vi "Wait.vi"() -> ()   [LabVIEW 2018]
uses:
  Framework/Robot Global Data.vi
panel:
  in  "Time":dbl
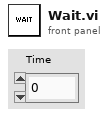
[diagram p1: front panel]
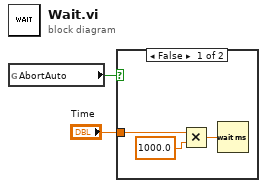
[diagram p0: block diagram]
diagram:
  n1 = global read "Robot Global Data.vi" "AbortAuto"() -> (w2:bool)
  n2 = case shown="False" w2 {
    tunnel: "Time" -> [w3 _]
    frame False {
      n3 = Multiply(x=w3, y=1000.0) -> (x*y=w5:dbl)
      n4 = Wait (ms)(milliseconds to wait=w5) -> ()  [unwired: 1 out]
    }
    frame True {
    }
  }
